vi "Set Ref.vi"(4 "Name":string, 6 "Name Msg":string, 8 "error in":errorcluster, 9 "Name Library File Path":path, 10 "Project:Active Project":refnum<vi>) -> (0 "error out":errorcluster, 2 "Ref":T1)   [LabVIEW 2025, in "_Msg Rescript.lvlib" / "_Msg Rescript.lvclass"]
uses:
  _Msg Rescript.lvclass
  Ref.ctl
  <vilib>/Utility/traverseref.llb/TRef TravTarget.ctl
  _Msg Rescript.lvclass/_Msg Rescript.ctl
  Poly VIs.ctl
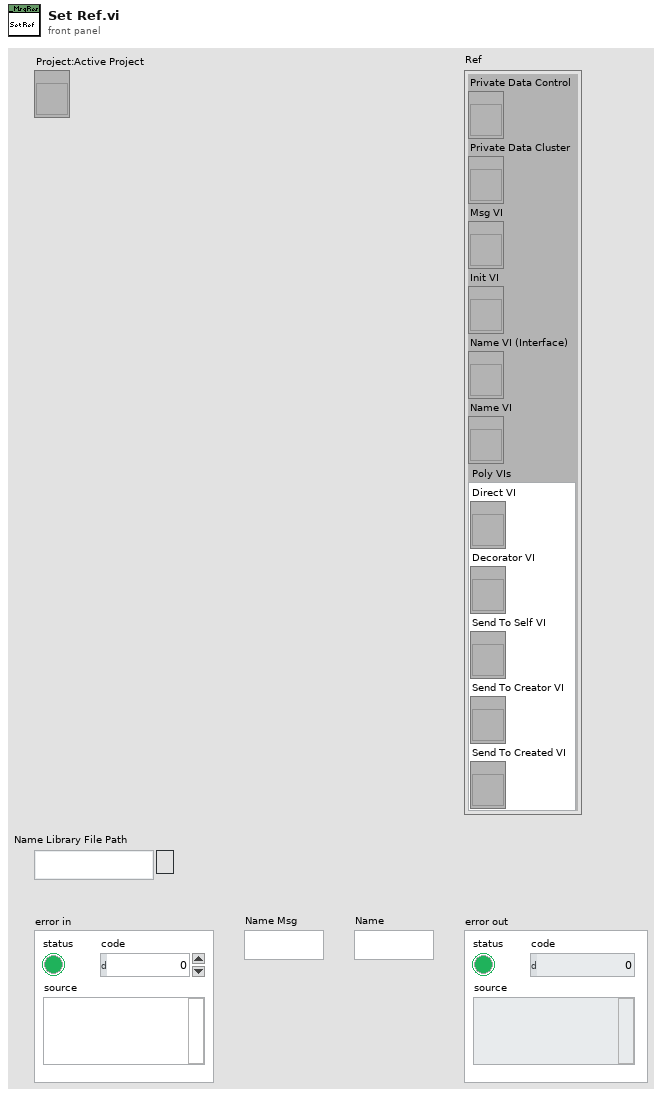
[diagram p1: front panel]
types:
  T1 = typedef "_Msg Rescript.lvlib/_Msg Rescript.lvclass/Ref.ctl" = cluster{"Private Data Control":refnum<vi>, "Private Data Cluster":refnum<vi>, "Msg VI":refnum<vi>, "Init VI":refnum<vi>, "Name VI (Interface)":refnum<vi>, "Name VI":refnum<vi>, "Poly VIs":T2}
  T2 = typedef "_Msg Rescript.lvlib/_Msg Rescript.lvclass/Poly VIs.ctl" = cluster{"Direct VI":refnum<vi>, "Decorator VI":refnum<vi>, "Send To Self VI":refnum<vi>, "Send To Creator VI":refnum<vi>, "Send To Created VI":refnum<vi>}
  T3 = typedef "TRef TravTarget.ctl" = enum16{"FP", "BD", "Other"}
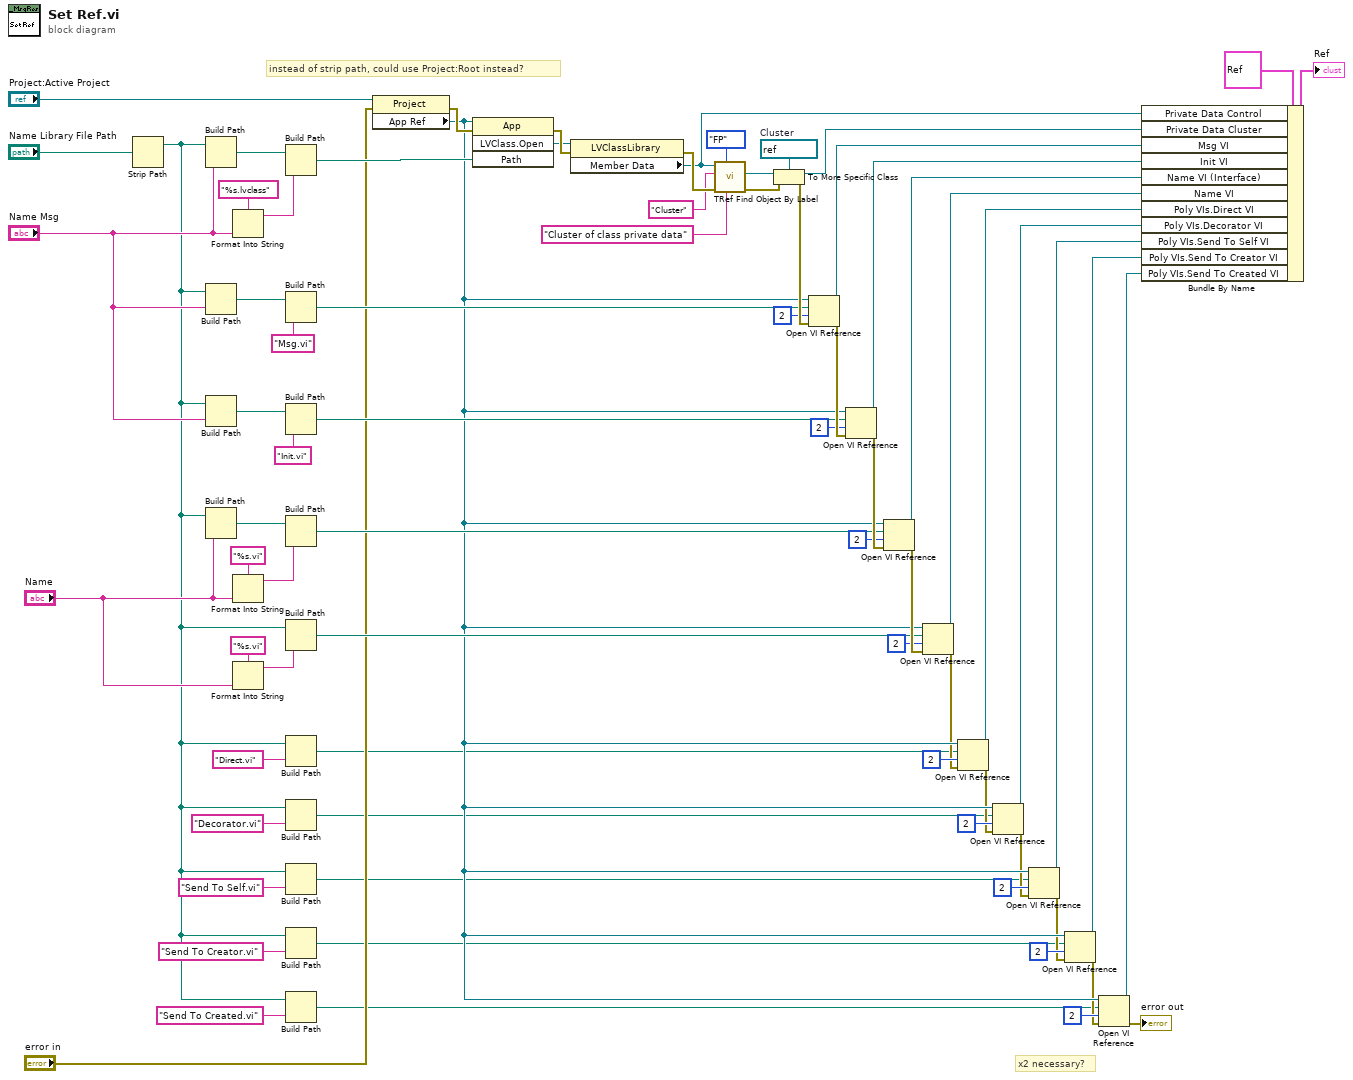
[diagram p0: block diagram]
diagram:
  w68 = refnum<vi> refnum  # Cluster
  # "instead of strip path, could use Project:Root instead?"
  # "x2 necessary?"
  n1 = Strip Path(path="Name Library File Path") -> (stripped path=w11:path)  [unwired: 1 out]
  n2 = Build Path(base path=w11, name or relative path="Name Msg") -> (appended path=w62:path)
  n3 = Build Path(base path=w11, name or relative path="Name Msg") -> (appended path=w55:path)
  n4 = Build Path(base path=w11, name or relative path="Name Msg") -> (appended path=w54:path)
  n5 = Build Path(base path=w11, name or relative path="Name") -> (appended path=w58:path)
  n6 = Format Into String(format string="%s.lvclass", "Name Msg") -> (resulting string=w60:string)  [unwired: 2 in, 1 out]
  n7 = Format Into String(format string="%s.vi", "Name") -> (resulting string=w57:string)  [unwired: 2 in, 1 out]
  n8 = Format Into String(format string="%s.vi", "Name") -> (resulting string=w48:string)  [unwired: 2 in, 1 out]
  n9 = Build Path(base path=w62, name or relative path=w60) -> (appended path=w61:path)
  n10 = Build Path(base path=w55, name or relative path="Msg.vi" ("format string")) -> (appended path=w51:path)
  n11 = Build Path(base path=w54, name or relative path="Init.vi" ("format string")) -> (appended path=w50:path)
  n12 = Build Path(base path=w58, name or relative path=w57) -> (appended path=w46:path)
  n13 = Build Path(base path=w11, name or relative path=w48) -> (appended path=w47:path)
  n14 = Build Path(base path=w11, name or relative path="Direct.vi" ("format string")) -> (appended path=w5:path)
  n15 = Build Path(base path=w11, name or relative path="Decorator.vi" ("format string")) -> (appended path=w4:path)
  n16 = Build Path(base path=w11, name or relative path="Send To Self.vi" ("format string")) -> (appended path=w3:path)
  n17 = Build Path(base path=w11, name or relative path="Send To Creator.vi" ("format string")) -> (appended path=w2:path)
  n18 = Build Path(base path=w11, name or relative path="Send To Created.vi" ("format string")) -> (appended path=w1:path)
  n19 = property class="Project"(reference="Project:Active Project", error in="error in") -> (error out=w72:errorcluster, "App Ref"=w23:refnum<vi>)  [unwired: 1 out]
  n20 = invoke class="App" method="LVClass.Open"(reference=w23, error in=w72, "Path"=w61) -> (error out=w70:errorcluster, "LVClass.Open"=w63:refnum<vi>)  [unwired: 1 in, 2 out]
  n21 = property class="LVClassLibrary"(reference=w63, error in=w70) -> (error out=w76:errorcluster, "Member Data"=w29:refnum<vi>)  [unwired: 1 out]
  n22 = call <vilib>:"TRef Find Object By Label.vi"("Label"="Cluster of class private data" ("Class Name"), "Traverse Target"=TRef_TravTarget."FP", "error in (no error)"=w76, "Class Name"="Cluster", "VI Ref"=w29) -> ("error out"=w69:errorcluster, "Found Obj Ref"=w67:refnum<vi>)  [unwired: 3 in, 2 out]
  n23 = To More Specific Class(target class=w68, reference=w67, error in=w69) -> (specific class reference=w34:refnum<vi>, error out=w71:errorcluster)
  n24 = Open VI Reference(application reference (local)=w23, vi path=w51, options=2, error in (no error)=w71) -> (vi reference=w35:refnum<vi>, error out=w75:errorcluster)  [unwired: 2 in]
  n25 = Open VI Reference(application reference (local)=w23, vi path=w50, options=2, error in (no error)=w75) -> (vi reference=w36:refnum<vi>, error out=w74:errorcluster)  [unwired: 2 in]
  n26 = Open VI Reference(application reference (local)=w23, vi path=w46, options=2, error in (no error)=w74) -> (vi reference=w37:refnum<vi>, error out=w73:errorcluster)  [unwired: 2 in]
  n27 = Open VI Reference(application reference (local)=w23, vi path=w47, options=2, error in (no error)=w73) -> (vi reference=w38:refnum<vi>, error out=w17:errorcluster)  [unwired: 2 in]
  n28 = Open VI Reference(application reference (local)=w23, vi path=w5, options=2, error in (no error)=w17) -> (vi reference=w22:refnum<vi>, error out=w16:errorcluster)  [unwired: 2 in]
  n29 = Open VI Reference(application reference (local)=w23, vi path=w4, options=2, error in (no error)=w16) -> (vi reference=w21:refnum<vi>, error out=w15:errorcluster)  [unwired: 2 in]
  n30 = Open VI Reference(application reference (local)=w23, vi path=w3, options=2, error in (no error)=w15) -> (vi reference=w20:refnum<vi>, error out=w14:errorcluster)  [unwired: 2 in]
  n31 = Open VI Reference(application reference (local)=w23, vi path=w2, options=2, error in (no error)=w14) -> (vi reference=w19:refnum<vi>, error out=w13:errorcluster)  [unwired: 2 in]
  n32 = Open VI Reference(application reference (local)=w23, vi path=w1, options=2, error in (no error)=w13) -> (vi reference=w18:refnum<vi>, error out=→"error out":errorcluster)  [unwired: 2 in]
  n33 = Bundle By Name(cluster=T1 {"Private Data Control"=refnum, "Private Data Cluster"=refnum, "Msg VI"=refnum, "Init VI"=refnum, "Name VI (Interface)"=refnum, "Name VI"=refnum, "Poly VIs"={"Direct VI"=refnum, "Decorator VI"=refnum, "Send To Self VI"=refnum, "Send To Creator VI"=refnum, "Send To Created VI"=refnum}} ("Ref"), "Private Data Control"=w29, "Private Data Cluster"=w34, "Msg VI"=w35, "Init VI"=w36, "Name VI (Interface)"=w37, "Name VI"=w38, "Poly VIs.Direct VI"=w22, "Poly VIs.Decorator VI"=w21, "Poly VIs.Send To Self VI"=w20, "Poly VIs.Send To Creator VI"=w19, "Poly VIs.Send To Created VI"=w18) -> (→"Ref":T1)
